vi "NanotecSMCPD.get axis onOff.vi"(0 "i ref in":refnum<vi>, 1 "axis":i32, 3 "ms timeout (10000)":i32=10000, 5 "error in (no error)":errorcluster) -> (14 "i ref out":refnum<vi>, 15 "onOff":bool, 17 "timed out":bool, 19 "error out":errorcluster)   [LabVIEW 2014, in "NanotecSMCPD.lvlib"]
doc: "Checks, if the axis is switched on."
uses:
  NanotecSMCPD.lvlib
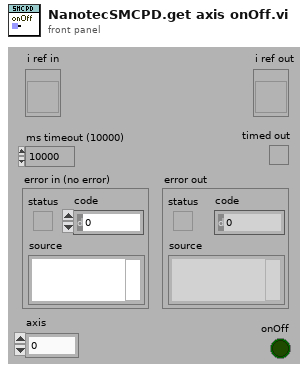
[diagram p1: front panel]
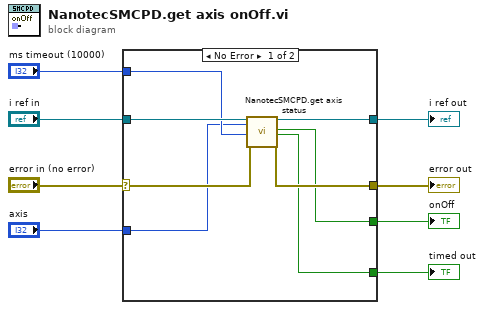
[diagram p0: block diagram]
diagram:
  n1 = case shown="No Error" "error in (no error)" {
    selector: "error in (no error)" -> [w14 w17]
    tunnel: "ms timeout (10000)" -> [w12 _]
    tunnel: "i ref in" -> [w16 w18]
    tunnel: [w13 w17] -> w5
    tunnel: "axis" -> [w11 _]
    tunnel: [w15 w18] -> w3
    tunnel: [w10 _] -> w2
    tunnel: [w9 _] -> w1
    frame No Error {
      n2 = call "NanotecSMCPD.get axis status.vi"("i ref in"=w16, "axis"=w11, "ms timeout (10000)"=w12, "error in (no error)"=w14) -> ("i ref out"=w15:refnum<vi>, "motorOn"=w10:bool, "timed out"=w9:bool, "error out"=w13:errorcluster)  [unwired: 11 in, 1 out]
    }
    frame Error {
    }
  }
  "error out" <- w5
  "i ref out" <- w3
  "timed out" <- w1
  "onOff" <- w2
